vi "GUI modeling.vi"() -> ()   [LabVIEW 2023]
panel:
  out "Target22 21":bool
  out "Ring22 21":bool
  out "Target22 20":bool
  out "Ring22 20":bool
  out "Target22 19":bool
  out "Ring22 19":bool
  out "Target22 18":bool
  out "Ring22 18":bool
  out "Target22 17":bool
  out "Ring22 17":bool
  out "Target22 16":bool
  out "Ring22 16":bool
  out "Target22 15":bool
  out "Ring22 15":bool
  out "Target22 14":bool
  out "Ring22 14":bool
  out "Target22 13":bool
  out "Ring22 13":bool
  out "Target22 12":bool
  out "Ring22 12":bool
  out "Target18":bool
  out "Ring18":bool
  out "Target22 5":bool
  out "Ring22 5":bool
  out "Target22 4":bool
  out "Ring22 4":bool
  out "Target22 11":bool
  out "Ring22 11":bool
  out "Target22 10":bool
  out "Ring22 10":bool
  out "Target22 3":bool
  out "Ring22 3":bool
  out "Target22 9":bool
  out "Ring22 9":bool
  out "Target22 8":bool
  out "Ring22 8":bool
  out "Target22 7":bool
  out "Ring22 7":bool
  out "Target22 6":bool
  out "Ring22 6":bool
  out "Target20":bool
  out "Ring20":bool
  out "Target21":bool
  out "Ring21":bool
  out "Target22":bool
  out "Ring22":bool
  out "Target17":bool
  out "Ring17":bool
  out "Target19":bool
  out "Ring19":bool
  out "Target22 2":bool
  out "Ring22 2":bool
  # "AprilTag not detected"
  # "AprilTag detected"
  # "Position unavailable"
  # "Position available"
  # "Position selected"
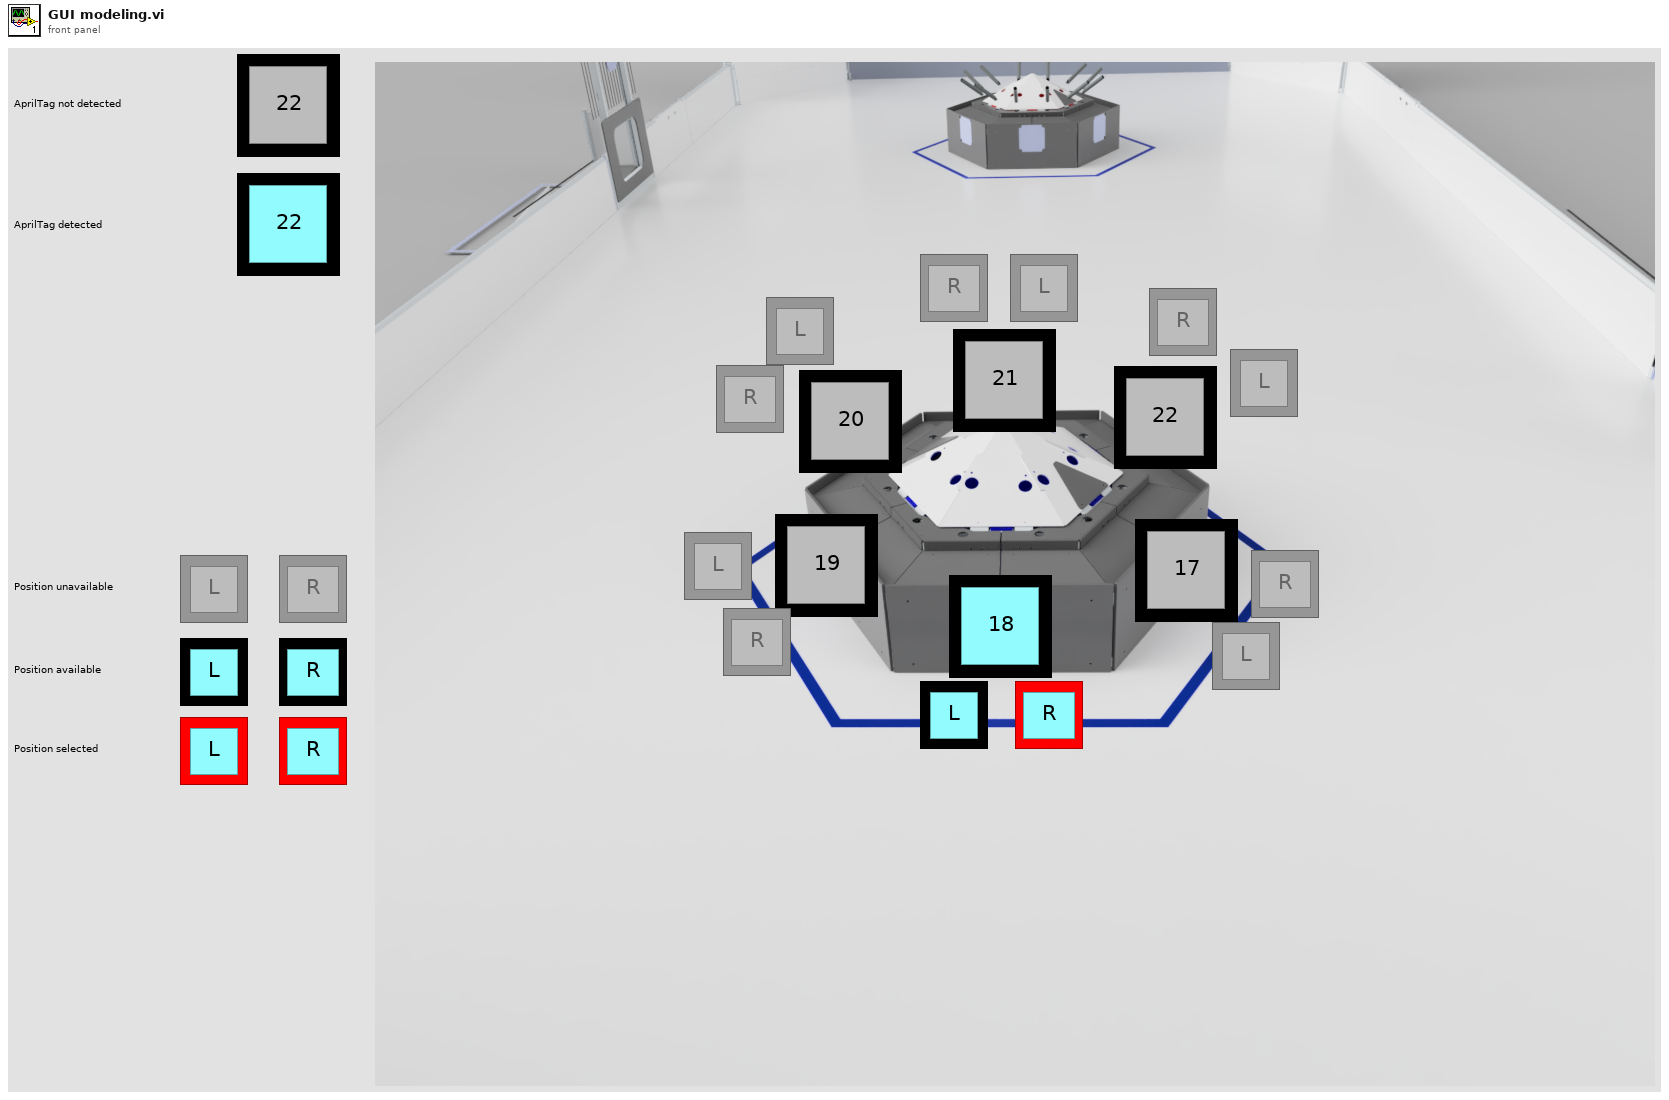
[diagram p1: front panel]
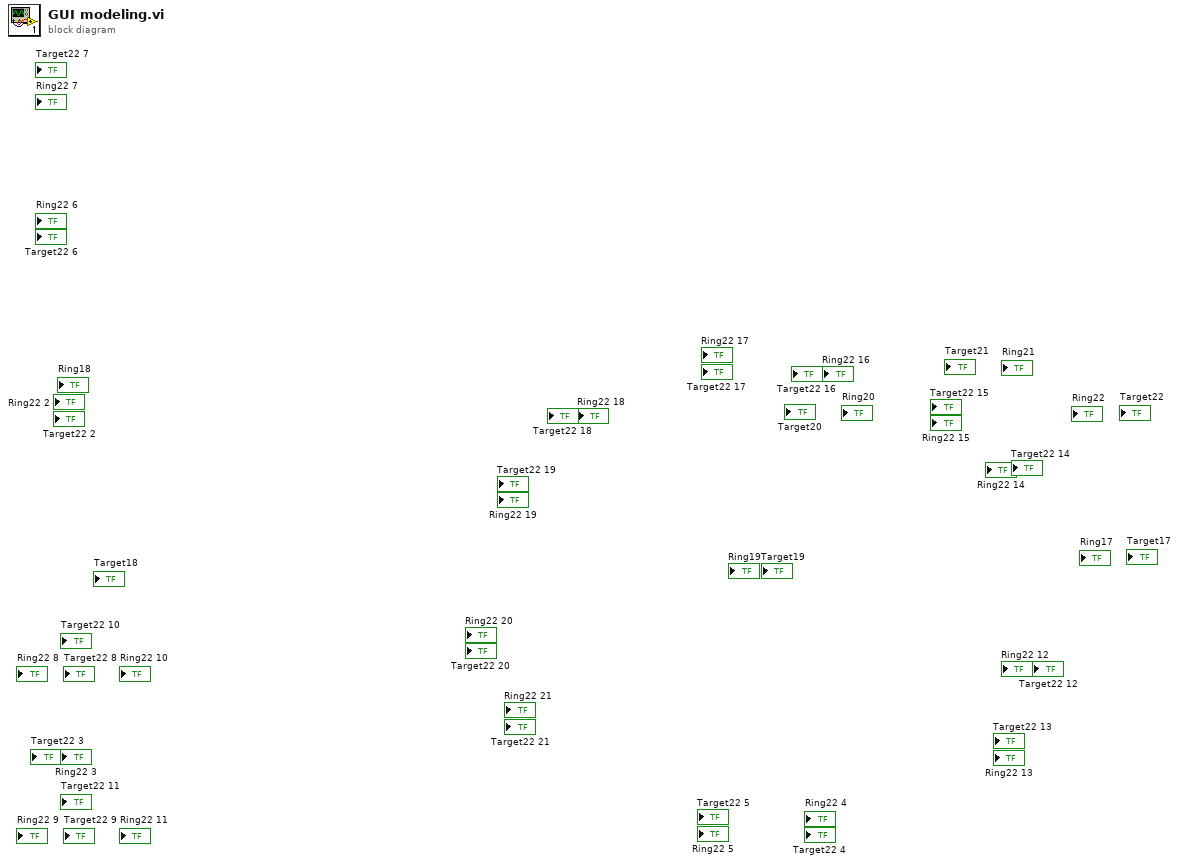
[diagram p0: block diagram]
diagram:
